vi "FTW-Actor-Child-PoisonPill.vi"(0 "FTW-ActorInstance In":refnum<class "FTW-ActorInstance.lvclass">, 5 "Connector Name":string, 9 "Timeout":i32=100 format="%dmsec", 11 "error in":errorcluster, 12 "Remove If No Error":bool=TRUE caption="Remove If No Error or Timeout") -> (4 "FTW-ActorInstance Out":refnum<class "FTW-ActorInstance.lvclass">, 6 "Response Header":string, 8 "Response Body":string, 10 "Timed out?":bool, 14 "Roundtrip Time":dbl format="%.6fsec", 15 "error out":errorcluster)   [LabVIEW 2015, in "FTW-ActorInstance.lvclass"]
uses:
  FTW-ActorInstance.lvclass
  Connector/FTW-ActorConnector.lvclass
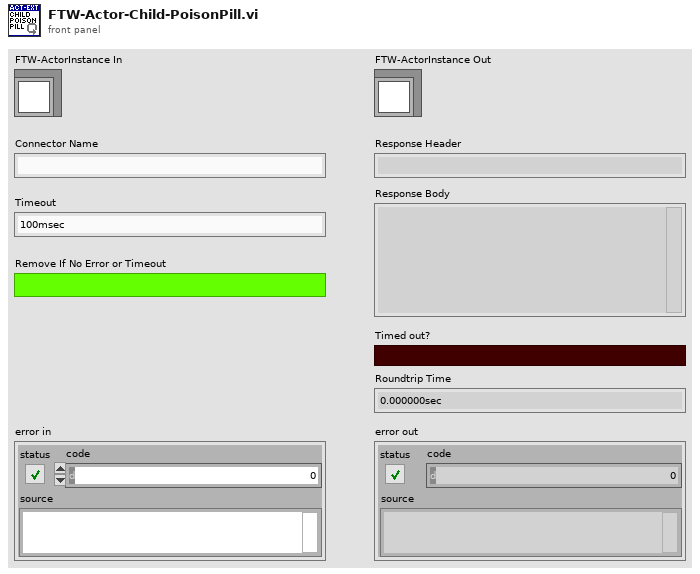
[diagram p1: front panel]
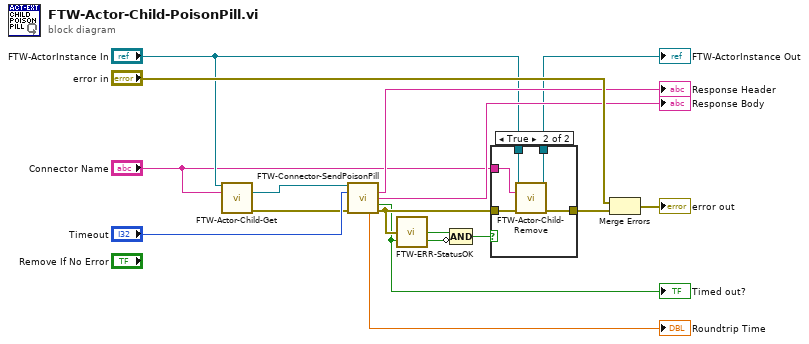
[diagram p0: block diagram]
diagram:
  n1 = call "FTW-Actor-Child-Get.vi"("FTW-ActorInstance In"="FTW-ActorInstance In", "Connector Name"="Connector Name") -> ("FTW Actor Connector"=w10:refnum<class "FTW-ActorConnector.lvclass">, "error out"=w11:errorcluster)  [unwired: 11 in, 1 out]
  n2 = call-dynamic "FTW-Connector-SendPoisonPill.vi"("FTW Actor Connector"=w10, "Timeout"="Timeout", "error in"=w11) -> ("Response Header"=→"Response Header":string, "Response Body"=→"Response Body":string, "Timed out?"=w1:bool, "Roundtrip Time"=→"Roundtrip Time":dbl, "error out"=w4:errorcluster)  [unwired: 7 in, 1 out]
  "Timed out?" <- w1
  n3 = call "FTW-ERR-StatusOK.vi"("error to check"=w4) -> ("Status OK?"=w3:bool)
  n4 = Compound Arithmetic op=AND(w3, invert w1) -> (w2:bool)
  n5 = case shown="True" w2 {
    tunnel: w4 -> [w17 w23]
    tunnel: [w17 w22] -> w8
    tunnel: "FTW-ActorInstance In" -> [w18 w21]
    tunnel: [w18 w20] -> w6
    tunnel: "Connector Name" -> [_ w19]
    frame False {
    }
    frame True {
      n6 = call "FTW-Actor-Child-Remove.vi"("FTW-ActorInstance In"=w21, "Connector Name"=w19, "error in"=w23) -> ("FTW-ActorInstance Out"=w20:refnum<class "FTW-ActorInstance.lvclass">, "error out"=w22:errorcluster)  [unwired: 11 in]
    }
  }
  "FTW-ActorInstance Out" <- w6
  n7 = Merge Errors("error in", w8) -> (→"error out":errorcluster)
